vi "Ventilador2.vi"() -> ()   [LabVIEW 2019]
uses:
  <vilib>/Analysis/polynomials.llb/Polynomial Roots (DBL).vi
  <vilib>/Analysis/NI_AALPro.lvlib
panel:
  in  "Vertical Pointer Slide":dbl
  out "Aquisição pressão respiratória":dbl(graph)
  out "Válvula expiração":dbl(graph)
  in  "Pausa inspiração":dbl
  in  "Limite pressão inspiratória":dbl
  in  "OK Button":bool
  in  "Root 3":dbl
  in  "Root 2":dbl
  in  "Root 1":dbl
  in  "Incremento":dbl
  in  "Fluxo inicial":dbl
  in  "STOP":bool=TRUE
  out "Tempos de inspirações possíveis":cdb[](array[numeric])
  out "Tempo do ciclo respiratório":u32(graph)
  out "Válvula Inspiração":dbl(graph)
  in  "stop":bool
  in  "Tempo de respiração":dbl
  in  "Proporção Inspiração/respiração":string(combo)
  in  "Tempo corrido":dbl
  in  "Tipo de ventilação":string(combo)
  in  "Tipo de ciclo":string(combo)
  in  "Volume corrente":dbl
  in  "Tempo expiratório":dbl
  in  "Tempo inspiratório":dbl
  out "Fluxo respiratório medido":dbl
  in  "Frequência respiratória":dbl
  in  "Forma de onda":string(combo)
  in  "Fluxo respiratório set point":dbl
  # "rpm"
  # "(s)"
  # "(cmH2O)"
  # "(cmH2O)"
  # "(s)"
  # "(s)"
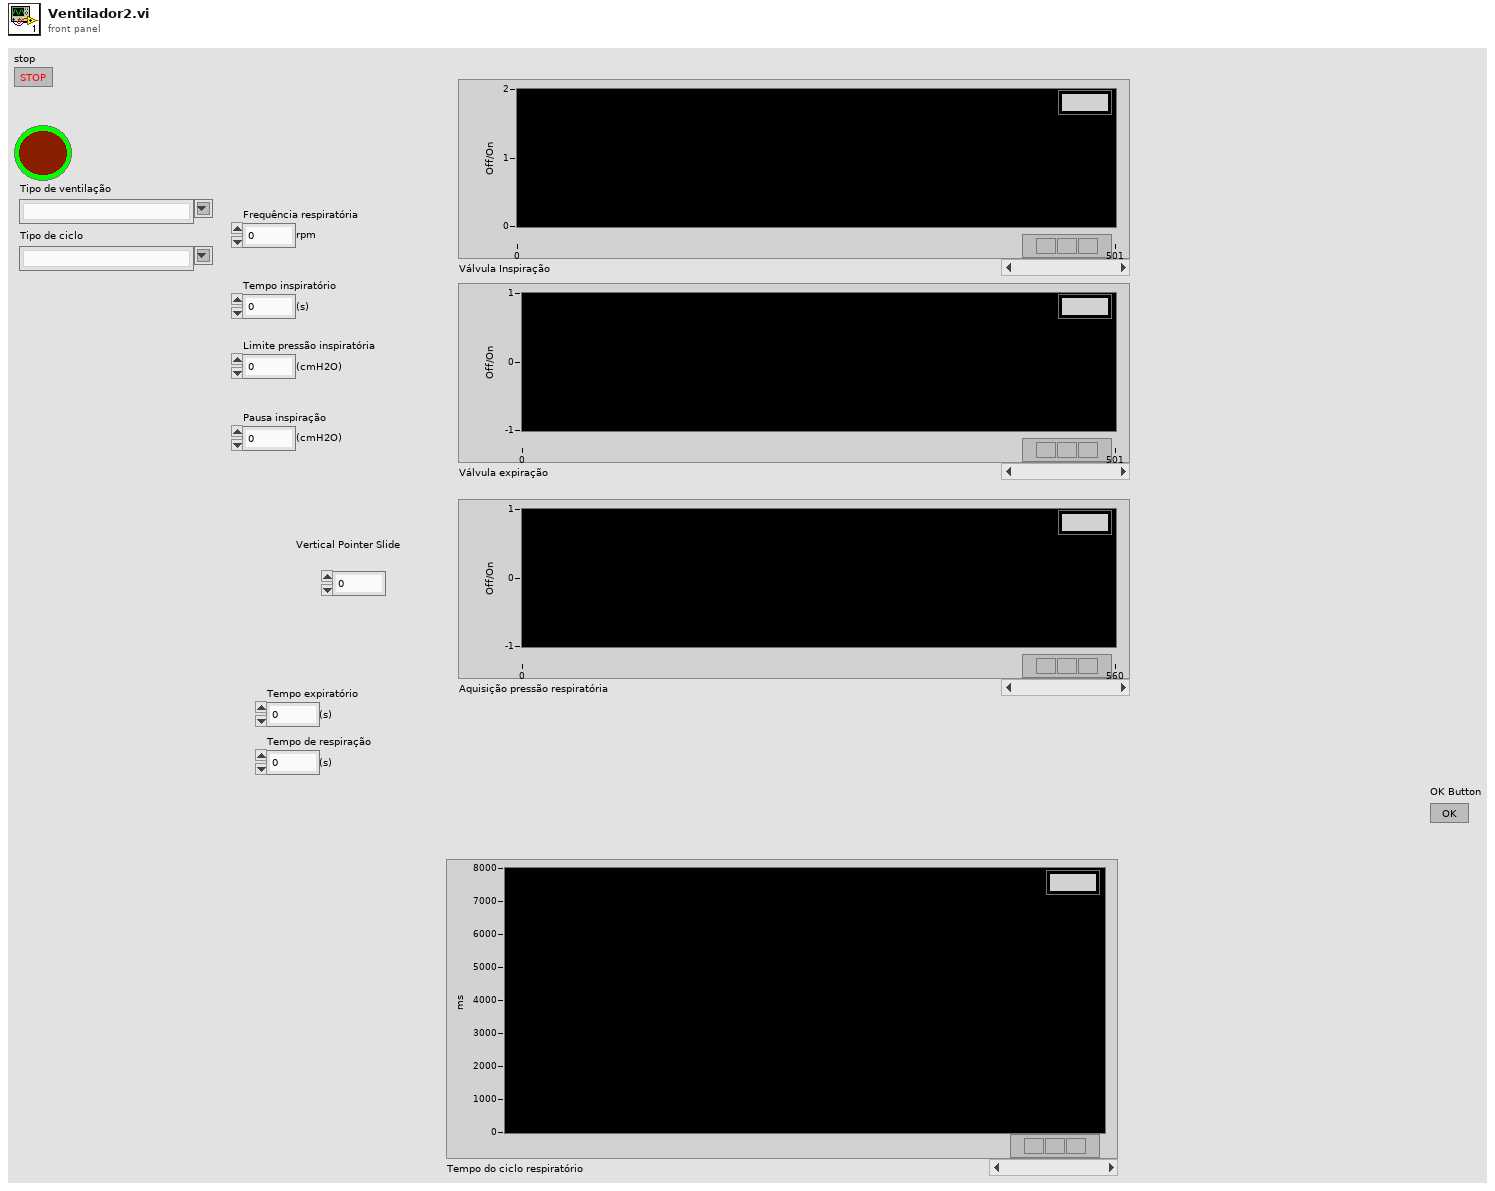
[diagram p1: front panel]
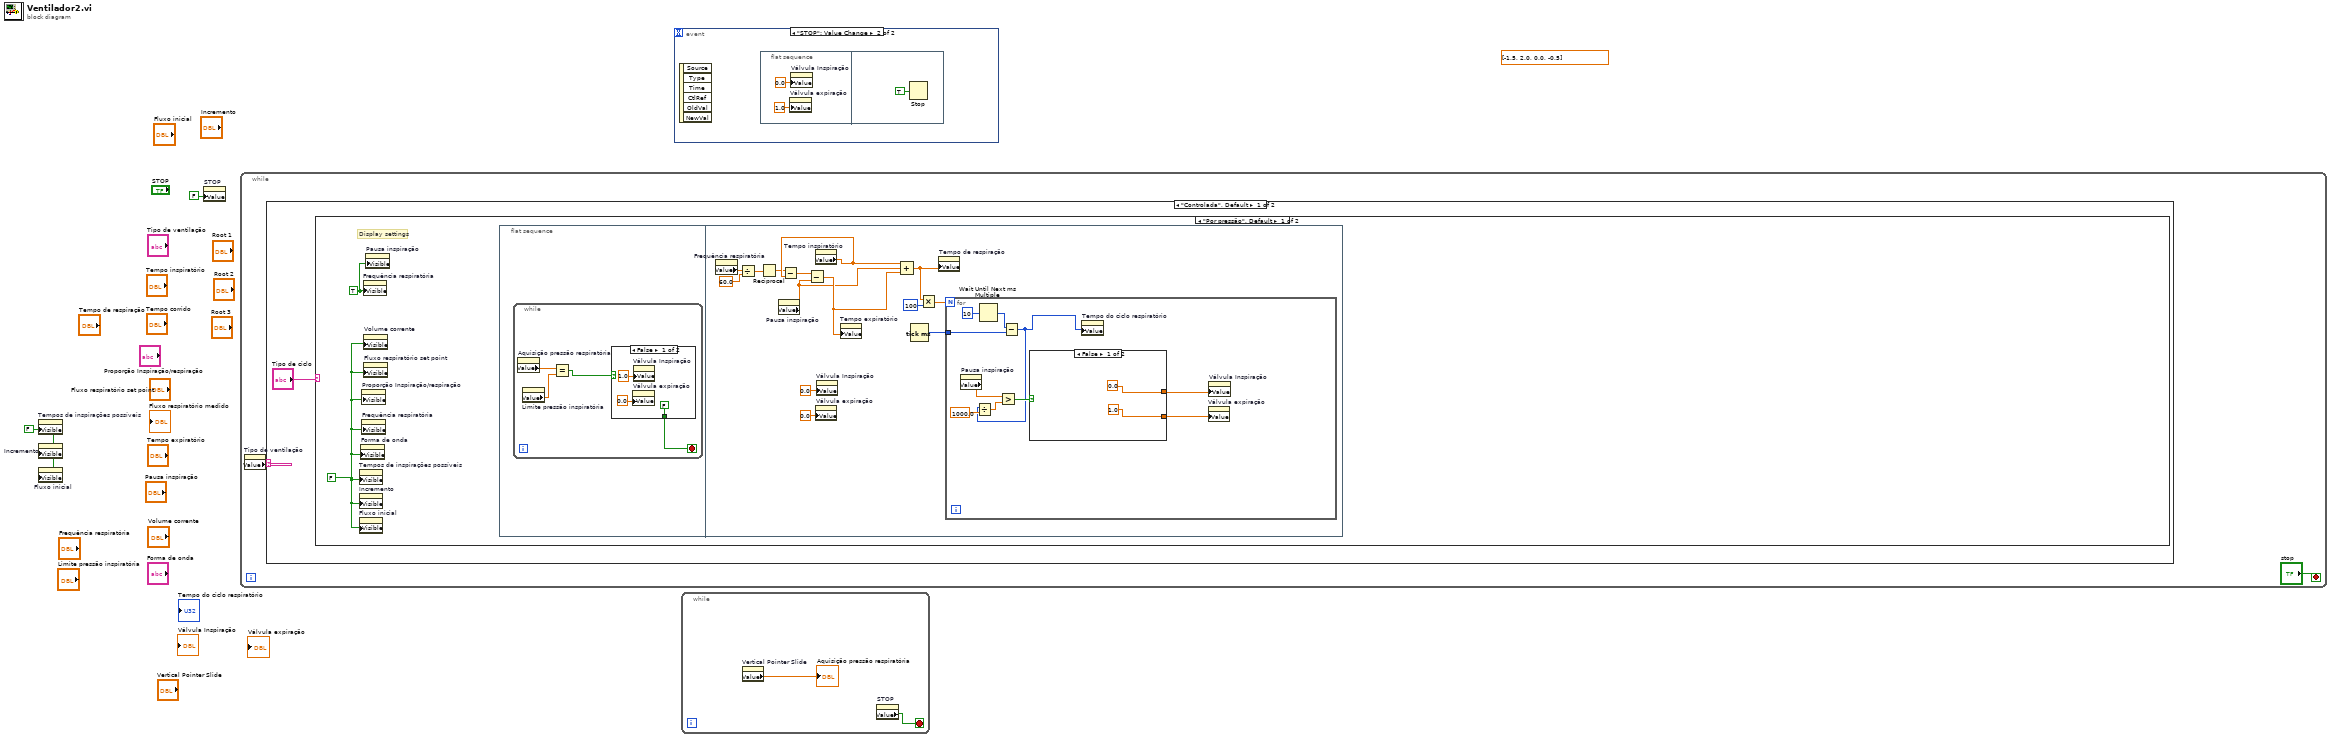
[diagram p0: block diagram]
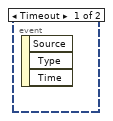
[diagram p2: hidden frame]
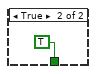
[diagram p3: hidden frame]
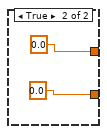
[diagram p4: hidden frame]
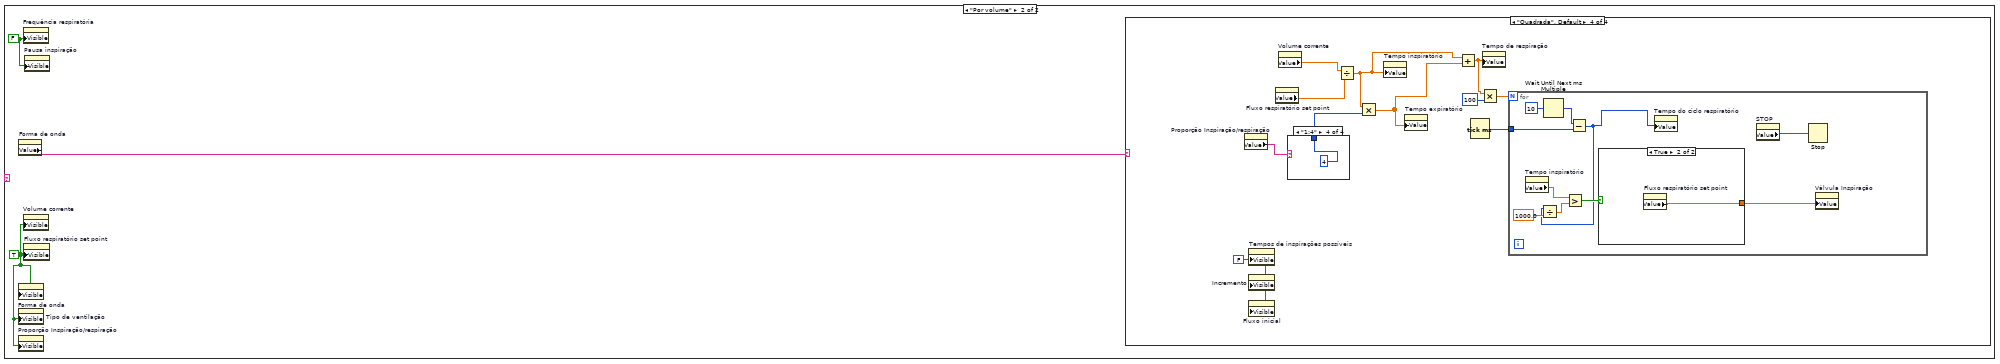
[diagram p5: hidden frame]
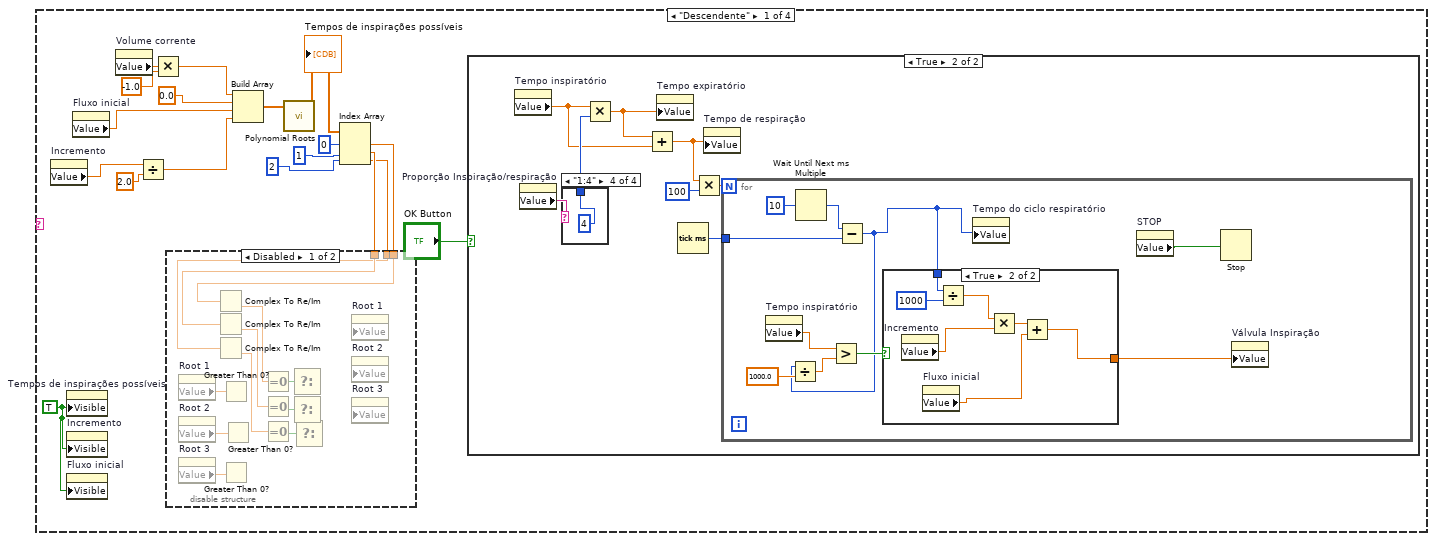
[diagram p6: hidden frame]
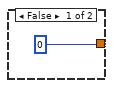
[diagram p9: hidden frame]
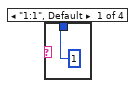
[diagram p10: hidden frame]
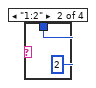
[diagram p11: hidden frame]
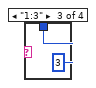
[diagram p12: hidden frame]
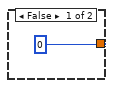
[diagram p15: hidden frame]
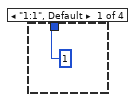
[diagram p16: hidden frame]
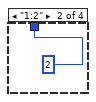
[diagram p17: hidden frame]
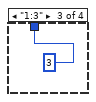
[diagram p18: hidden frame]
diagram:
  w1 = FALSE ("Visible")
  (unwired) dbl[] [-1.5, 2.0, 0.0, -0.5] ("P(x)")
  n1 = property on="Tempos de inspirações possíveis" class="Arr (strict)"("Visible"=w1) -> ()  [unwired: 2 in, 2 out]
  n2 = property on="Incremento" class="DigNum (strict)"("Visible"=w1) -> ()  [unwired: 2 in, 2 out]
  n3 = property on="Fluxo inicial" class="DigNum (strict)"("Visible"=w1) -> ()  [unwired: 2 in, 2 out]
  n4 = property on="STOP" class="Bool (strict)"("Value"=FALSE ("STOP")) -> ()  [unwired: 2 in, 2 out]
  n5 = while {
    stop <- "stop" stop-if-true
    n6 = property on="Tipo de ventilação" class="CmbBox"() -> ("Value"=w4:string)  [unwired: 2 in, 2 out]
    n7 = case shown="\"Controlada\", Default" w4 {
      frame "Controlada", Default {
        n8 = case shown="\"Por pressão\", Default" "Tipo de ciclo" {
          frame "Por pressão", Default {
            w6 = TRUE ("Visible")
            w7 = FALSE ("Visible")
            # "Display settings"
            n9 = property on="Tempos de inspirações possíveis" class="Arr (strict)"("Visible"=w7) -> ()  [unwired: 2 in, 2 out]
            n10 = property on="Incremento" class="DigNum (strict)"("Visible"=w7) -> ()  [unwired: 2 in, 2 out]
            n11 = property on="Fluxo inicial" class="DigNum (strict)"("Visible"=w7) -> ()  [unwired: 2 in, 2 out]
            n12 = property on="Forma de onda" class="CmbBox"("Visible"=w7) -> ()  [unwired: 2 in, 2 out]
            n13 = property on="Proporção Inspiração/respiração" class="CmbBox"("Visible"=w7) -> ()  [unwired: 2 in, 2 out]
            n14 = property on="Frequência respiratória" class="DigNum (strict)"("Visible"=w7) -> ()  [unwired: 2 in, 2 out]
            n15 = property on="Frequência respiratória" class="DigNum (strict)"("Visible"=w6) -> ()  [unwired: 2 in, 2 out]
            n16 = property on="Volume corrente" class="DigNum (strict)"("Visible"=w7) -> ()  [unwired: 2 in, 2 out]
            n17 = property on="Fluxo respiratório set point" class="DigNum (strict)"("Visible"=w7) -> ()  [unwired: 2 in, 2 out]
            n18 = property on="Pausa inspiração" class="DigNum (strict)"("Visible"=w6) -> ()  [unwired: 2 in, 2 out]
            n19 = flat-sequence {
              frame #0 {
                n20 = while {
                  stop <- w10 stop-if-true
                  n21 = property on="Aquisição pressão respiratória" class="WFChart (strict)"() -> ("Value"=w8:dbl)  [unwired: 2 in, 2 out]
                  n22 = property on="Limite pressão inspiratória" class="DigNum (strict)"() -> ("Value"=w11:dbl)  [unwired: 2 in, 2 out]
                  n23 = Equal?(x=w8, y=w11) -> (x = y?=w9:bool)
                  n24 = case shown="False" w9 {
                    tunnel: [FALSE TRUE] -> w10
                    frame False {
                      n25 = property on="Válvula expiração" class="WFChart (strict)"("Value"=0.0 ("Válvula expiração")) -> ()  [unwired: 2 in, 2 out]
                      n26 = property on="Válvula Inspiração" class="WFChart (strict)"("Value"=1.0 ("Válvula Inspiração")) -> ()  [unwired: 2 in, 2 out]
                    }
                    frame True {
                    }
                  }
                }
              }
              frame #1 {
                n27 = property on="Frequência respiratória" class="DigNum (strict)"() -> ("Value"=w22:dbl)  [unwired: 2 in, 2 out]
                n28 = Divide(x=w22, y=60.0) -> (x/y=w23:dbl)
                n29 = Reciprocal(x=w23) -> (1/x=w24:dbl)
                n30 = property on="Pausa inspiração" class="DigNum (strict)"() -> ("Value"=w27:dbl)  [unwired: 2 in, 2 out]
                n31 = property on="Tempo inspiratório" class="DigNum (strict)"() -> ("Value"=w26:dbl)  [unwired: 2 in, 2 out]
                n32 = Subtract(x=w24, y=w26) -> (x-y=w25:dbl)
                n33 = Subtract(x=w25, y=w27) -> (x-y=w28:dbl)
                n34 = property on="Válvula expiração" class="WFChart (strict)"("Value"=0.0 ("Válvula expiração")) -> ()  [unwired: 2 in, 2 out]
                n35 = property on="Válvula Inspiração" class="WFChart (strict)"("Value"=0.0 ("Válvula Inspiração")) -> ()  [unwired: 2 in, 2 out]
                n36 = property on="Tempo expiratório" class="DigNum (strict)"("Value"=w28) -> ()  [unwired: 2 in, 2 out]
                n37 = Compound Arithmetic op=ADD(w26, w27, w28) -> (w29:dbl)
                n38 = Tick Count (ms)() -> (millisecond timer value=w20:u32)
                n39 = Multiply(x=w29, y=100) -> (x*y=w21:dbl)
                n40 = property on="Tempo de respiração" class="DigNum (strict)"("Value"=w29) -> ()  [unwired: 2 in, 2 out]
                n41 = for {
                  N: w21 -> [_]
                  tunnel: w20 -> [w37]
                  n42 = property on="Pausa inspiração" class="DigNum (strict)"() -> ("Value"=w35:dbl)  [unwired: 2 in, 2 out]
                  n43 = Wait Until Next ms Multiple(millisecond multiple=u32 10) -> (millisecond timer value=w39:u32)
                  n44 = Subtract(x=w39, y=w37) -> (x-y=w32:u32)
                  n45 = Divide(x=w32, y=1000.0) -> (x/y=w34:dbl)
                  n46 = Greater?(x=w35, y=w34) -> (0:w36:bool)
                  n47 = case shown="False" w36 {
                    tunnel: [0.0 ("Válvula Inspiração") 0.0 ("y")] -> w31
                    tunnel: [1.0 ("Válvula expiração") 0.0 ("y")] -> w30
                    frame False {
                    }
                    frame True {
                    }
                  }
                  n48 = property on="Tempo do ciclo respiratório" class="WFChart (strict)"("Value"=w32) -> ()  [unwired: 2 in, 2 out]
                  n49 = property on="Válvula expiração" class="WFChart (strict)"("Value"=w30) -> ()  [unwired: 2 in, 2 out]
                  n50 = property on="Válvula Inspiração" class="WFChart (strict)"("Value"=w31) -> ()  [unwired: 2 in, 2 out]
                }
              }
            }
          }
          frame "Por volume" {
            w44 = FALSE ("Visible")
            w45 = TRUE ("Visible")
            n51 = property on="Forma de onda" class="CmbBox"("Visible"=w45) -> ()  [unwired: 2 in, 2 out]
            n52 = property on="Tipo de ventilação" class="CmbBox"("Visible"=w45) -> ()  [unwired: 2 in, 2 out]
            n53 = property on="Proporção Inspiração/respiração" class="CmbBox"("Visible"=w45) -> ()  [unwired: 2 in, 2 out]
            n54 = property on="Forma de onda" class="CmbBox"() -> ("Value"=w46:string)  [unwired: 2 in, 2 out]
            n55 = property on="Frequência respiratória" class="DigNum (strict)"("Visible"=w44) -> ()  [unwired: 2 in, 2 out]
            n56 = property on="Volume corrente" class="DigNum (strict)"("Visible"=w45) -> ()  [unwired: 2 in, 2 out]
            n57 = property on="Fluxo respiratório set point" class="DigNum (strict)"("Visible"=w45) -> ()  [unwired: 2 in, 2 out]
            n58 = property on="Pausa inspiração" class="DigNum (strict)"("Visible"=w44) -> ()  [unwired: 2 in, 2 out]
            n59 = case shown="\"Quadrada\", Default" w46 {
              frame "Descendente" {
                w47 = TRUE ("Visible")
                n60 = property on="Incremento" class="DigNum (strict)"() -> ("Value"=w63:dbl)  [unwired: 2 in, 2 out]
                n61 = property on="Tempos de inspirações possíveis" class="Arr (strict)"("Visible"=w47) -> ()  [unwired: 2 in, 2 out]
                n62 = property on="Incremento" class="DigNum (strict)"("Visible"=w47) -> ()  [unwired: 2 in, 2 out]
                n63 = property on="Fluxo inicial" class="DigNum (strict)"("Visible"=w47) -> ()  [unwired: 2 in, 2 out]
                n64 = property on="Fluxo inicial" class="DigNum (strict)"() -> ("Value"=w52:dbl)  [unwired: 2 in, 2 out]
                n65 = property on="Volume corrente" class="DigNum (strict)"() -> ("Value"=w62:dbl)  [unwired: 2 in, 2 out]
                n66 = Divide(x=w63, y=2.0) -> (x/y=w51:dbl)
                n67 = Multiply(x=w62, y=-1.0) -> (x*y=w54:dbl)
                n68 = Build Array(w54, 0.0 ("element"), w52, w51) -> (w50:dbl[])
                n69 = call-poly <vilib>:"Polynomial Roots.vi"("P(x)"=w50) -> ("Roots"=w64:cdb[])  [unwired: 9 in, 1 out]
                "Tempos de inspirações possíveis" <- w64
                n70 = Index Array(array=w64, index #1=0 ("index"), index #2=1 ("index"), index #3=2 ("index")) -> (element #1=w49:cdb, element #2=w56:cdb, element #3=w55:cdb)
                n71 = disable-structure shown="Disabled" {
                  disable-tunnel: w56 -> [w76 _]
                  disable-tunnel: w55 -> [w75 _]
                  disable-tunnel: w49 -> [w74 _]
                  frame Disabled {
                    n72 = property on="Root 1" class="DigNum (strict)"() -> ("Value"=w73:dbl)  [unwired: 2 in, 2 out]
                    n73 = property on="Root 2" class="DigNum (strict)"() -> ("Value"=w72:dbl)  [unwired: 2 in, 2 out]
                    n74 = property on="Root 3" class="DigNum (strict)"() -> ("Value"=w71:dbl)  [unwired: 2 in, 2 out]
                    n75 = Complex To Re/Im(x + iy=w74) -> (y=w68:dbl)  [unwired: 1 out]
                    n76 = Complex To Re/Im(x + iy=w76) -> (y=w69:dbl)  [unwired: 1 out]
                    n77 = Complex To Re/Im(x + iy=w75) -> (y=w70:dbl)  [unwired: 1 out]
                    n78 = Greater Than 0?(x=w73) -> ()  [unwired: 1 out]
                    n79 = Greater Than 0?(x=w71) -> ()  [unwired: 1 out]
                    n80 = Greater Than 0?(x=w72) -> ()  [unwired: 1 out]
                    n81 = Equal To 0?(x=w68) -> (x = 0?=w67:bool)
                    n82 = Equal To 0?(x=w69) -> (x = 0?=w66:bool)
                    n83 = Equal To 0?(x=w70) -> (x = 0?=w65:bool)
                    n84 = Select(s=w67) -> ()  [unwired: 2 in, 1 out]
                    n85 = Select(s=w66) -> ()  [unwired: 2 in, 1 out]
                    n86 = Select(s=w65) -> ()  [unwired: 2 in, 1 out]
                    n87 = property on="Root 1" class="DigNum (strict)" props=["Value"]() -> ()  [unwired: 3 in, 2 out]
                    n88 = property on="Root 2" class="DigNum (strict)" props=["Value"]() -> ()  [unwired: 3 in, 2 out]
                    n89 = property on="Root 3" class="DigNum (strict)" props=["Value"]() -> ()  [unwired: 3 in, 2 out]
                  }
                  frame Enabled {
                  }
                }
                n90 = case shown="True" "OK Button" {
                  frame False {
                  }
                  frame True {
                    n91 = property on="Tempo inspiratório" class="DigNum (strict)"() -> ("Value"=w78:dbl)  [unwired: 2 in, 2 out]
                    n92 = property on="Proporção Inspiração/respiração" class="CmbBox"() -> ("Value"=w84:string)  [unwired: 2 in, 2 out]
                    n93 = case shown="\"1:4\"" w84 {
                      tunnel: [1 2 3 4] -> w80
                      frame "1:1", Default {
                      }
                      frame "1:2" {
                      }
                      frame "1:3" {
                      }
                      frame "1:4" {
                      }
                    }
                    n94 = Multiply(x=w78, y=w80) -> (x*y=w79:dbl)
                    n95 = Add(x=w79, y=w78) -> (x+y=w77:dbl)
                    n96 = property on="Tempo expiratório" class="DigNum (strict)"("Value"=w79) -> ()  [unwired: 2 in, 2 out]
                    n97 = Tick Count (ms)() -> (millisecond timer value=w83:u32)
                    n98 = Multiply(x=w77, y=100) -> (x*y=w82:dbl)
                    n99 = property on="Tempo de respiração" class="DigNum (strict)"("Value"=w77) -> ()  [unwired: 2 in, 2 out]
                    n100 = for {
                      N: w82 -> [_]
                      tunnel: w83 -> [w92]
                      n101 = property on="Tempo inspiratório" class="DigNum (strict)"() -> ("Value"=w90:dbl)  [unwired: 2 in, 2 out]
                      n102 = Wait Until Next ms Multiple(millisecond multiple=u32 10) -> (millisecond timer value=w94:u32)
                      n103 = Subtract(x=w94, y=w92) -> (x-y=w86:u32)
                      n104 = Divide(x=w86, y=1000.0) -> (x/y=w89:dbl)
                      n105 = Greater?(x=w90, y=w89) -> (0:w91:bool)
                      n106 = case shown="True" w91 {
                        tunnel: [0 w97] -> w85
                        tunnel: w86 -> [_ w102]
                        frame False {
                        }
                        frame True {
                          n107 = property on="Incremento" class="DigNum (strict)"() -> ("Value"=w99:dbl)  [unwired: 2 in, 2 out]
                          n108 = property on="Fluxo inicial" class="DigNum (strict)"() -> ("Value"=w96:dbl)  [unwired: 2 in, 2 out]
                          n109 = Divide(x=w102, y=u32 1000) -> (x/y=w100:dbl)
                          n110 = Multiply(x=w100, y=w99) -> (x*y=w98:dbl)
                          n111 = Add(x=w98, y=w96) -> (x+y=w97:dbl)
                        }
                      }
                      n112 = property on="Tempo do ciclo respiratório" class="WFChart (strict)"("Value"=w86) -> ()  [unwired: 2 in, 2 out]
                      n113 = property on="STOP" class="Bool (strict)"() -> ("Value"=w87:bool)  [unwired: 2 in, 2 out]
                      n114 = Stop(stop? (T)=w87) -> ()
                      n115 = property on="Válvula Inspiração" class="WFChart (strict)"("Value"=w85) -> ()  [unwired: 2 in, 2 out]
                    }
                  }
                }
              }
              frame "Ascendente" {
              }
              frame "Sinusoidal" {
              }
              frame "Quadrada", Default {
                w107 = FALSE ("Visible")
                n116 = property on="Proporção Inspiração/respiração" class="CmbBox"() -> ("Value"=w115:string)  [unwired: 2 in, 2 out]
                n117 = property on="Tempos de inspirações possíveis" class="Arr (strict)"("Visible"=w107) -> ()  [unwired: 2 in, 2 out]
                n118 = property on="Incremento" class="DigNum (strict)"("Visible"=w107) -> ()  [unwired: 2 in, 2 out]
                n119 = property on="Fluxo inicial" class="DigNum (strict)"("Visible"=w107) -> ()  [unwired: 2 in, 2 out]
                n120 = property on="Fluxo respiratório set point" class="DigNum (strict)"() -> ("Value"=w117:dbl)  [unwired: 2 in, 2 out]
                n121 = property on="Volume corrente" class="DigNum (strict)"() -> ("Value"=w116:dbl)  [unwired: 2 in, 2 out]
                n122 = case shown="\"1:4\"" w115 {
                  tunnel: [1 2 3 4] -> w114
                  frame "1:1", Default {
                  }
                  frame "1:2" {
                  }
                  frame "1:3" {
                  }
                  frame "1:4" {
                  }
                }
                n123 = Divide(x=w116, y=w117) -> (x/y=w111:dbl)
                n124 = Multiply(x=w111, y=w114) -> (x*y=w110:dbl)
                n125 = property on="Tempo inspiratório" class="DigNum (strict)"("Value"=w111) -> ()  [unwired: 2 in, 2 out]
                n126 = property on="Tempo expiratório" class="DigNum (strict)"("Value"=w110) -> ()  [unwired: 2 in, 2 out]
                n127 = Add(x=w111, y=w110) -> (x+y=w109:dbl)
                n128 = Tick Count (ms)() -> (millisecond timer value=w113:u32)
                n129 = Multiply(x=w109, y=100) -> (x*y=w112:dbl)
                n130 = property on="Tempo de respiração" class="DigNum (strict)"("Value"=w109) -> ()  [unwired: 2 in, 2 out]
                n131 = for {
                  N: w112 -> [_]
                  tunnel: w113 -> [w125]
                  n132 = property on="Tempo inspiratório" class="DigNum (strict)"() -> ("Value"=w123:dbl)  [unwired: 2 in, 2 out]
                  n133 = Wait Until Next ms Multiple(millisecond multiple=u32 10) -> (millisecond timer value=w127:u32)
                  n134 = Subtract(x=w127, y=w125) -> (x-y=w120:u32)
                  n135 = Divide(x=w120, y=1000.0) -> (x/y=w122:dbl)
                  n136 = Greater?(x=w123, y=w122) -> (0:w124:bool)
                  n137 = case shown="True" w124 {
                    tunnel: [0 w129] -> w119
                    frame False {
                    }
                    frame True {
                      n138 = property on="Fluxo respiratório set point" class="DigNum (strict)"() -> ("Value"=w129:dbl)  [unwired: 2 in, 2 out]
                    }
                  }
                  n139 = property on="Tempo do ciclo respiratório" class="WFChart (strict)"("Value"=w120) -> ()  [unwired: 2 in, 2 out]
                  n140 = property on="STOP" class="Bool (strict)"() -> ("Value"=w118:bool)  [unwired: 2 in, 2 out]
                  n141 = Stop(stop? (T)=w118) -> ()
                  n142 = property on="Válvula Inspiração" class="WFChart (strict)"("Value"=w119) -> ()  [unwired: 2 in, 2 out]
                }
              }
            }
          }
        }
      }
      frame "Expontânea/Assistida" {
      }
    }
  }
  n143 = event shown="[1] \"STOP\": Value Change" {
    selector: _ -> [_ _]
    dyn-events: _ -> [_ _]
    timeout: _ -> [_ _]
    event Timeout {
      n144 = event-data() -> ()  [unwired: 1 in, 3 out]
    }
    event "STOP": Value Change {
      n145 = event-data() -> ()  [unwired: 1 in, 6 out]
      n146 = flat-sequence {
        frame #0 {
          n147 = property on="Válvula expiração" class="WFChart (strict)"("Value"=1.0 ("Válvula expiração")) -> ()  [unwired: 2 in, 2 out]
          n148 = property on="Válvula Inspiração" class="WFChart (strict)"("Value"=0.0 ("Válvula Inspiração")) -> ()  [unwired: 2 in, 2 out]
        }
        frame #1 {
          n149 = Stop(stop? (T)=TRUE) -> ()
        }
      }
    }
  }
  n150 = while {
    stop <- w138 stop-if-true
    n151 = property on="Vertical Pointer Slide" class="DigNum (strict)"() -> ("Value"=→"Aquisição pressão respiratória":dbl)  [unwired: 2 in, 2 out]
    n152 = property on="STOP" class="Bool (strict)"() -> ("Value"=w138:bool)  [unwired: 2 in, 2 out]
  }
